vi "LHF.DB.Mongo.Collection.Core.Insert.vi"(8 "error in (no error)":errorcluster, 9 "collectionName":string, 10 "BsonDocument":refnum<k24>, 11 "LHF.DB.Mongo in":refnum<class "LHF.DB.Mongo.lvclass">) -> (0 "error out":errorcluster, 2 "BsonDocument out":refnum<k24>, 3 "LHF.DB.Mongo out":refnum<class "LHF.DB.Mongo.lvclass">)   [LabVIEW 2013, in "LHF.DB.Mongo.lvclass"]
uses:
  LHF.DB.Mongo.lvclass
  C:/Users/schim/Desktop/Projetos/LabVIEW-MongoDB/src/Driver/MongoDB.Bson.dll
  Driver/MongoDB.Bson.dll
  C:/Users/schim/Desktop/Projetos/LabVIEW-MongoDB/src/Driver/MongoDB.Driver.dll
  Driver/MongoDB.Driver.dll
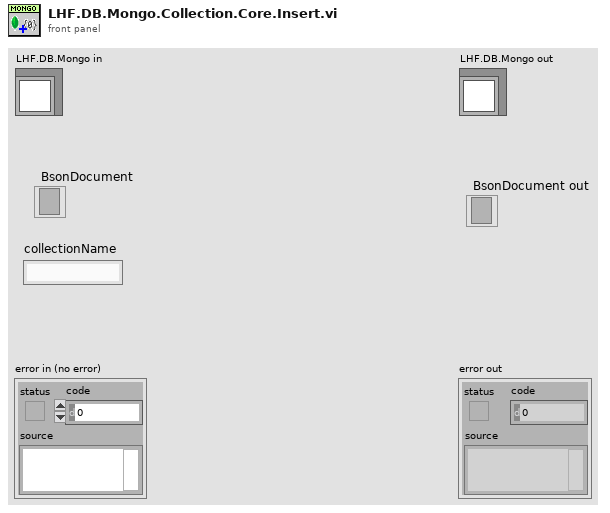
[diagram p1: front panel]
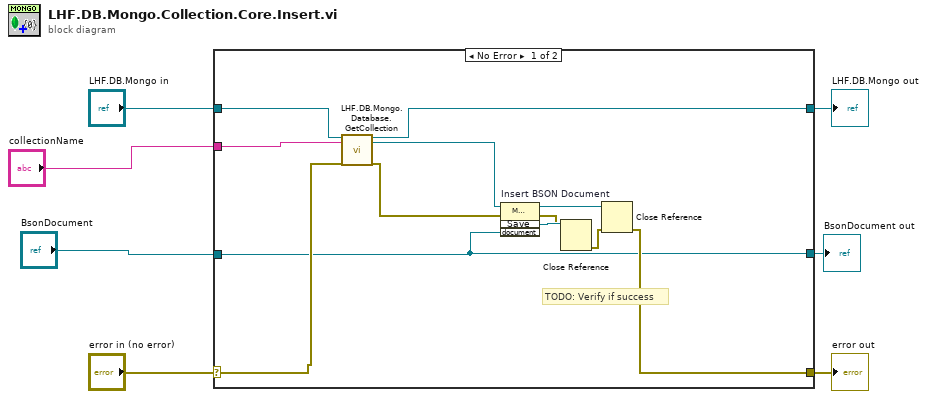
[diagram p0: block diagram]
diagram:
  n1 = case shown="No Error" "error in (no error)" {
    selector: "error in (no error)" -> [w18 w22]
    tunnel: [w12 w22] -> w6
    tunnel: [w14 w21] -> w4
    tunnel: "LHF.DB.Mongo in" -> [w15 w21]
    tunnel: "collectionName" -> [w19 _]
    tunnel: "BsonDocument" -> [w11 w20]
    tunnel: [w11 w20] -> w1
    frame No Error {
      # "TODO: Verify if success"
      n2 = call "LHF.DB.Mongo.Database.GetCollection.vi"("LHF.DB.Mongo in"=w15, "collectionName"=w19, "error in (no error)"=w18) -> ("LHF.DB.Mongo in"=w14:refnum<class "LHF.DB.Mongo.lvclass">, "MongoCollection"=w17:refnum<k24>, "error out"=w16:errorcluster)  [unwired: 14 in]
      n3 = invoke on="Insert BSON Document" class="MongoCollection`1[[MongoDB.Bson" method="Save"(reference=w17, error in=w16, "document"=w11) -> (reference out=w13:refnum<k24>, error out=w9:errorcluster, "Save"=w10:refnum<k24>)  [unwired: 1 in, 1 out]
      n4 = Close Reference(reference=w10, error in (no error)=w9) -> (error out=w8:errorcluster)
      n5 = Close Reference(reference=w13, error in (no error)=w8) -> (error out=w12:errorcluster)
    }
    frame Error {
    }
  }
  "error out" <- w6
  "LHF.DB.Mongo out" <- w4
  "BsonDocument out" <- w1
